vi "Set Lock.vi"(10 "lock":refnum<k33>, 11 "Pointer in":refnum<class "Pointer.lvclass">) -> (3 "Pointer out":refnum<class "Pointer.lvclass">)   [LabVIEW 2016, in "Memory Manager.lvlib" / "Pointer.lvclass"]
uses:
  Pointer.lvclass
  Pointer.lvclass/Pointer.ctl
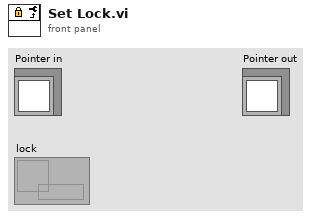
[diagram p1: front panel]
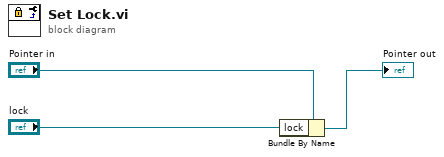
[diagram p0: block diagram]
diagram:
  n1 = Bundle By Name(cluster="Pointer in", "lock"="lock") -> (→"Pointer out":refnum<class "Pointer.lvclass">)
